vi "CircularBuffer.GenerateBufferSizeChangedEvent.vi"(8 "error in (no error)":errorcluster, 11 "CircularBuffer in":refnum<class "CircularBuffer.lvclass">) -> (0 "error out":errorcluster, 3 "CircularBuffer out":refnum<class "CircularBuffer.lvclass">)   [LabVIEW 2013, in "CircularBuffer.lvclass"]
uses:
  CircularBuffer.lvclass
  Typedefs/ValueChanged--EventData--Cluster.ctl
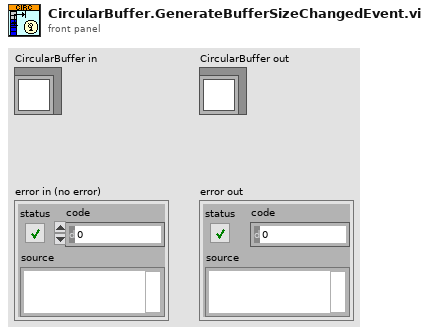
[diagram p1: front panel]
types:
  T1 = typedef "CircularBuffer.lvclass/ValueChanged--EventData--Cluster.ctl" = cluster{"BufferSize":i32}
  T2 = typedef "CircularBuffer.lvclass/PublicEvents--Cluster.ctl" = cluster{"Buffer Resize Event":refnum<user-event>}
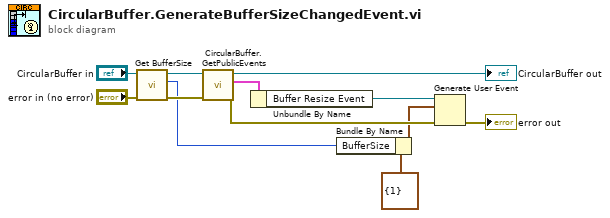
[diagram p0: block diagram]
diagram:
  n1 = call "Get BufferSize.vi"("error in (no error)"="error in (no error)", "CircularBuffer"="CircularBuffer in") -> ("error out"=w2:errorcluster, "BufferSize"=w1:i32, "CircularBuffer out"=w4:refnum<class "CircularBuffer.lvclass">)  [unwired: 7 in]
  n2 = call "CircularBuffer.GetPublicEvents.vi"("error in (no error)"=w2, "CircularBuffer"=w4) -> ("error out"=w10:errorcluster, "CircBuffer Public Events"=w9:T2, "CircularBuffer out"=→"CircularBuffer out":refnum<class "CircularBuffer.lvclass">)  [unwired: 7 in]
  n3 = Unbundle By Name(w9) -> ("Buffer Resize Event"=w6:refnum<user-event>)
  n4 = Bundle By Name(cluster=T1 {"BufferSize"=1} ("event data"), "BufferSize"=w1) -> (w8:T1)
  n5 = Generate User Event(user event=w6, event data cluster=w8, error in=w10) -> (error out=→"error out":errorcluster)  [unwired: 1 in, 1 out]
